vi "LogPodStateData.vi"(8 "Iterations between saves":i32=10, 9 "Iteration counter":i32, 10 "All Pod State Data":T1(array[cluster]), 11 "Datalog File Refnum in":refnum<k34>) -> (3 "Datalog File Refnum out":refnum<k34>)   [LabVIEW 2014]
uses:
  Variables/Default global.vi
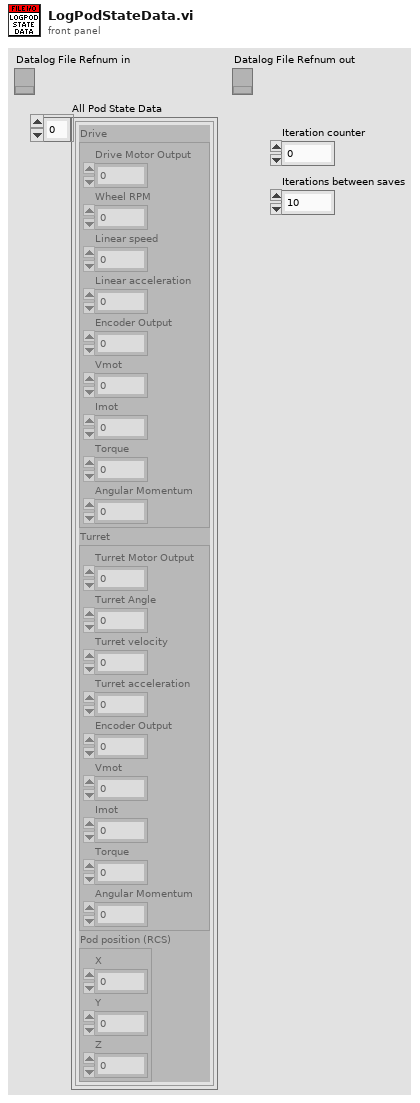
[diagram p1: front panel]
types:
  T1 = cluster{"Drive":cluster{"Drive Motor Output":dbl, "Wheel RPM":dbl, "Linear speed":dbl, "Linear acceleration":dbl, "Encoder Output":dbl, "Vmot":dbl, "Imot":dbl, "Torque":dbl, "Angular Momentum":dbl}, "Turret":cluster{"Turret Motor Output":dbl, "Turret Angle":dbl, "Turret velocity":dbl, "Turret acceleration":dbl, "Encoder Output":dbl, "Vmot":dbl, "Imot":dbl, "Torque":dbl, "Angular Momentum":dbl}, "Pod position (RCS)":cluster{"X":dbl, "Y":dbl, "Z":dbl}}[]
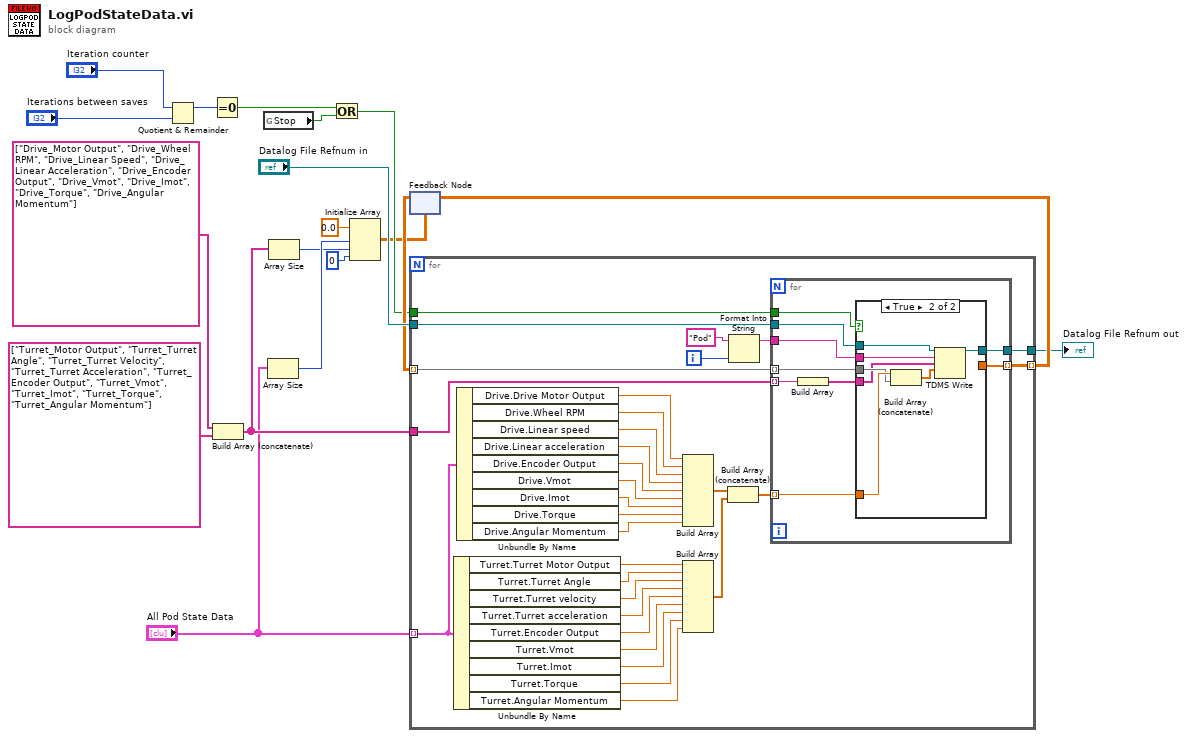
[diagram p0: block diagram]
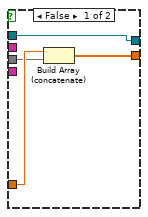
[diagram p2: hidden frame]
diagram:
  n1 = Quotient & Remainder(x="Iteration counter", y="Iterations between saves") -> (x-y*floor(x/y)=w14:i32)  [unwired: 1 out]
  n2 = Equal To 0?(x=w14) -> (x = 0?=w13:bool)
  n3 = Build Array (concatenate)(string[] ["Drive_Motor Output", "Drive_Wheel RPM", "Drive_Linear Speed", "Drive_Linear Acceleration", "Drive_Encoder Output", "Drive_Vmot", "Drive_Imot", "Drive_Torque", "Drive_Angular Momentum"] ("Array of Channels"), string[] ["Turret_Motor Output", "Turret_Turret Angle", "Turret_Turret Velocity", "Turret_Turret Acceleration", "Turret_Encoder Output", "Turret_Vmot", "Turret_Imot", "Turret_Torque", "Turret_Angular Momentum"] ("Array of Channels")) -> (w7:string[])
  n4 = global read "Default global.vi" "Stop"() -> (w12:bool)
  n5 = Array Size(array="All Pod State Data") -> (size(s)=w5:i32)
  n6 = Array Size(array=w7) -> (size(s)=w4:i32)
  n7 = Or(x=w13, y=w12) -> (x .or. y?=w10:bool)
  n8 = Initialize Array(0.0 ("element"), w5, w4, 0 ("dimension size")) -> (w1:dbl[][][])
  n9 = feedback #1(w1) -> (w17:dbl[][][])
  n10 = for {
    tunnel: "All Pod State Data" -> [w39] mode=indexing
    tunnel: "Datalog File Refnum in" -> [w33]
    tunnel: [w24] -> w18 mode=indexing
    tunnel: w17 -> [w23] mode=indexing
    tunnel: [w22] -> w11
    tunnel: w10 -> [w21]
    tunnel: w7 -> [w20]
    i -> [w38]
    n11 = Unbundle By Name(w39) -> ("Turret.Turret Motor Output"=w44:dbl, "Turret.Turret Angle"=w43:dbl, "Turret.Turret velocity"=w42:dbl, "Turret.Turret acceleration"=w41:dbl, "Turret.Encoder Output"=w40:dbl, "Turret.Vmot"=w37:dbl, "Turret.Imot"=w36:dbl, "Turret.Torque"=w31:dbl, "Turret.Angular Momentum"=w30:dbl)
    n12 = Unbundle By Name(w39) -> ("Drive.Drive Motor Output"=w45:dbl, "Drive.Wheel RPM"=w46:dbl, "Drive.Linear speed"=w47:dbl, "Drive.Linear acceleration"=w48:dbl, "Drive.Encoder Output"=w49:dbl, "Drive.Vmot"=w35:dbl, "Drive.Imot"=w34:dbl, "Drive.Torque"=w29:dbl, "Drive.Angular Momentum"=w28:dbl)
    n13 = Build Array(w45, w46, w47, w48, w49, w35, w34, w29, w28) -> (w26:dbl[])
    n14 = Build Array(w44, w43, w42, w41, w40, w37, w36, w31, w30) -> (w27:dbl[])
    n15 = Build Array (concatenate)(w26, w27) -> (w25:dbl[])
    n16 = Format Into String(initial string="Pod", w38) -> (resulting string=w32:string)  [unwired: 2 in, 1 out]
    n17 = for {
      tunnel: w33 -> [w53]
      tunnel: w32 -> [w54]
      tunnel: w25 -> [w59] mode=indexing
      tunnel: w20 -> [w58] mode=indexing
      tunnel: [w57] -> w24 mode=indexing
      tunnel: w23 -> [w56] mode=indexing
      tunnel: [w52] -> w22
      tunnel: w21 -> [w51]
      n18 = Build Array(w58) -> (w55:string[])
      n19 = case shown="True" w51 {
        tunnel: w59 -> [w63 w70]
        tunnel: [w62 _] -> w57
        tunnel: w56 -> [w61 w69]
        tunnel: w55 -> [_ w67]
        tunnel: w54 -> [_ w66]
        tunnel: w53 -> [w60 w65]
        tunnel: [w60 w64] -> w52
        frame False {
          n20 = Build Array (concatenate)(w63, w61) -> (w62:dbl[])
        }
        frame True {
          n21 = Build Array (concatenate)(w70, w69) -> (w68:dbl[])
          n22 = TDMS Write(0:w65, 5:w66, 7:w67, 9:w68) -> (4:w64:refnum<k34>)  [unwired: 2 in, 3 out]
        }
      }
    }
  }
  "Datalog File Refnum out" <- w11
  n23 = feedback-in #1(w18) -> ()
